vi "Get Generic Property.vi"(0 "SLSC Remote in":refnum<class "SLSC Remote.lvclass">, 1 "property type":T1, 5 "resources":string, 7 "property":refnum<k21>, 11 "error in (no error)":errorcluster) -> (4 "SLSC Remote out":refnum<class "SLSC Remote.lvclass">, 10 "property value":variant, 15 "error out":errorcluster)   [LabVIEW 2015, in "SLSC Remote.lvclass"]
uses:
  SLSC Remote.lvclass
  SLSC Interface Class/Property Type.ctl
  <vilib>/NI/i3 JSON/JSON Generation/Create Value Files/Create Value - Object.vi
  <vilib>/NI/i3 JSON/JSON Generation/Add Object Parameter Files/Add Object Parameter - String.vi
  <vilib>/NI/NI JSONRPC Server Framework/Classes/Server/Format Client Request (Auto-Increment).vi
  <vilib>/httpClient/POSTBuffer.vi
  <vilib>/NI/i3 JSON/JSON Parsing/Get Object Parameter Files/Get Object Parameter - Known Type.vi
  <vilib>/NI/NI JSONRPC Server Framework/Classes/Server/JSONRPC Server.lvclass
  <vilib>/NI/i3 JSON/i3-json.lvlib
  <vilib>/httpClient/LabVIEWHTTPClient.lvlib
  SLSC Interface Class/SLSC Interface.lvclass
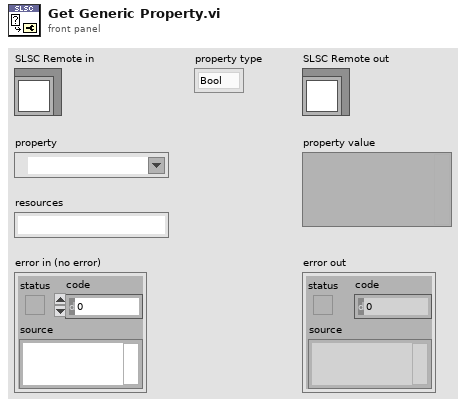
[diagram p1: front panel]
types:
  T1 = typedef "SLSC Interface.lvclass/Property Type.ctl" = enum16{"Bool", "DBL", "I32", "I64", "String", "U32", "U64", "1D Bool", "1D DBL", "1D I32", "1D I64", "1D String", "1D U32", "1D U64"}
  T2 = typedef "LabVIEWHTTPClient.lvlib/ClientHandle.ctl" = refnum<k1>
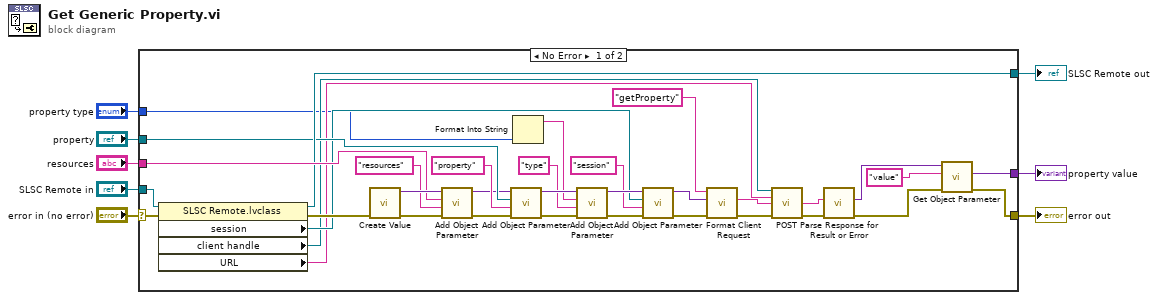
[diagram p0: block diagram]
diagram:
  n1 = case shown="No Error" "error in (no error)" {
    selector: "error in (no error)" -> [w36 w44]
    tunnel: "resources" -> [w42 _]
    tunnel: "SLSC Remote in" -> [w40 w45]
    tunnel: [w39 w45] -> w3
    tunnel: "property" -> [w37 _]
    tunnel: "property type" -> [w14 _]
    tunnel: [w9 w44] -> w2
    tunnel: [w11 _] -> w1
    frame No Error {
      n2 = property class="SLSC Remote.lvclass"(reference=w40, error in=w36) -> (reference out=w39:refnum<class "SLSC Remote.lvclass">, error out=w35:errorcluster, "session"=w25:refnum<k21>, "client handle"=w21:T2, "URL"=w20:string)
      n3 = call-poly <vilib>:"Create Value.vi"("error in (no error)"=w35) -> ("error out"=w34:errorcluster, "JSON Tree"=w43:variant)  [unwired: 9 in]
      n4 = call-poly <vilib>:"Add Object Parameter.vi"("error in (no error)"=w34, "Name"="resources", "String"=w42, "JSON Tree in (JSON Object)"=w43) -> ("error out"=w33:errorcluster, "JSON Tree out (JSON Object)"=w30:variant)  [unwired: 6 in]
      n5 = call-poly <vilib>:"Add Object Parameter.vi"("error in (no error)"=w33, "Name"="property", "String"=w37, "JSON Tree in (JSON Object)"=w30) -> ("error out"=w28:errorcluster, "JSON Tree out (JSON Object)"=w29:variant)  [unwired: 6 in]
      n6 = Format Into String(w14) -> (resulting string=w17:string)  [unwired: 3 in, 1 out]
      n7 = call-poly <vilib>:"Add Object Parameter.vi"("error in (no error)"=w28, "Name"="type" ("String"), "String"=w17, "JSON Tree in (JSON Object)"=w29) -> ("error out"=w26:errorcluster, "JSON Tree out (JSON Object)"=w27:variant)  [unwired: 6 in]
      n8 = call-poly <vilib>:"Add Object Parameter.vi"("error in (no error)"=w26, "Name"="session", "String"=w25, "JSON Tree in (JSON Object)"=w27) -> ("error out"=w22:errorcluster, "JSON Tree out (JSON Object)"=w23:variant)  [unwired: 6 in]
      n9 = call-poly <vilib>:"Format Client Request.vi"("error in (no error)"=w22, "params"=w23, "method"="getProperty") -> ("error out"=w19:errorcluster, "Request String"=w31:string)  [unwired: 7 in]
      n10 = call-poly <vilib>:"POST.vi"("client handle"=w21, "url"=w20, "buffer"=w31, "error in (no error)"=w19) -> ("body"=w16:string, "error out"=w15:errorcluster)  [unwired: 8 in, 2 out]
      n11 = call <vilib>:"Parse Response for Result or Error.vi"("error in"=w15, "Response String In"=w16) -> ("error out"=w10:errorcluster, "Result or Error Data"=w12:variant)  [unwired: 7 in, 1 out]
      n12 = call-poly <vilib>:"Get Object Parameter.vi"("error in (no error)"=w10, "Parameter Name"="value", "JSON Tree In (JSON Object)"=w12) -> ("error out"=w9:errorcluster, "Value"=w11:variant)  [unwired: 3 in, 4 out]
    }
    frame Error {
    }
  }
  "error out" <- w2
  "SLSC Remote out" <- w3
  "property value" <- w1
